vi "WB_Imp_WB10C_RGB_sub.vi"(2 "weights&Biases_cvs_file path":path=path "C:/Users/박원일/NEPL Dropbox/연구실 공용/뉴로모픽 과제/weights/weights_f_93.csv") -> (0 "W_10C(R)":i64[][](array[numeric]), 1 "B_10C(R)":i64[](array[numeric]), 3 "W_10C(B)":i64[][](array[numeric]), 4 "B_10C(B)":i64[](array[numeric]), 5 "W_10C(G)":i64[][](array[numeric]), 6 "B_10C(G)":i64[](array[numeric]))   [LabVIEW 2021]
uses:
  <vilib>/Utility/file.llb/Read Delimited Spreadsheet (DBL).vi
panel:
  in  "format (%.3f)":string="%.3f"
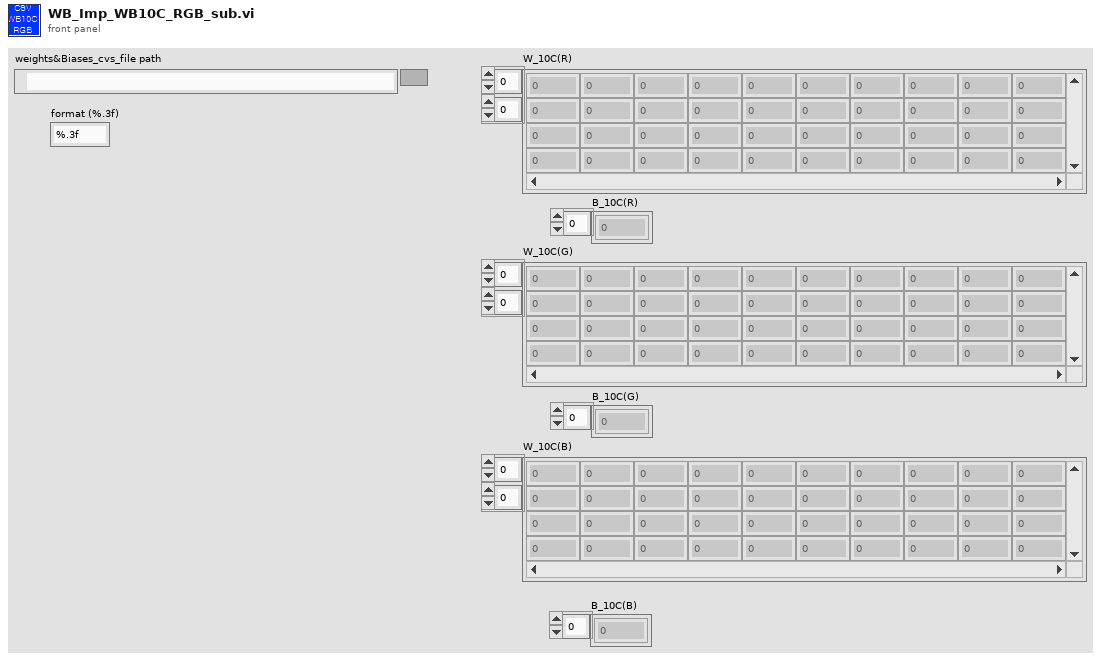
[diagram p1: front panel]
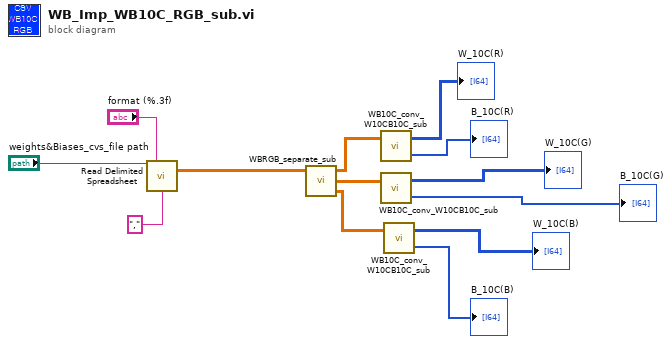
[diagram p0: block diagram]
diagram:
  n1 = call-poly <vilib>:"Read Delimited Spreadsheet.vi"("file path (dialog if empty)"="weights&Biases_cvs_file path", "format (%.3f)"="format (%.3f)", "delimiter (\\t)"="," ("delimiter (\\t)")) -> ("all rows"=w10:dbl[][])  [unwired: 7 in, 5 out]
  n2 = call "WBRGB_separate_sub.vi"("WB_RGB"=w10) -> ("WB_B"=w7:dbl[][], "WB_G"=w8:dbl[][], "WB_R"=w9:dbl[][])  [unwired: 2 in]
  n3 = call "WB10C_conv_W10CB10C_sub.vi"("WB_10C_input"=w9) -> ("B_10C"=→"B_10C(R)":i64[], "W_10C"=→"W_10C(R)":i64[][])  [unwired: 1 in]
  n4 = call "WB10C_conv_W10CB10C_sub.vi"("WB_10C_input"=w8) -> ("B_10C"=→"B_10C(G)":i64[], "W_10C"=→"W_10C(G)":i64[][])  [unwired: 1 in]
  n5 = call "WB10C_conv_W10CB10C_sub.vi"("WB_10C_input"=w7) -> ("B_10C"=→"B_10C(B)":i64[], "W_10C"=→"W_10C(B)":i64[][])  [unwired: 1 in]
